vi "Error Handling Core.vi"(8 "error in (no error)":errorcluster) -> (0 "error out":errorcluster)   [LabVIEW 2016, in "System.lvlib"]
doc: "This is the core VI for error logging.\nWhen the error occurred, this VI will sned abort event to other processes."
uses:
  System.lvlib
  Controls/Control_Data Functions.ctl
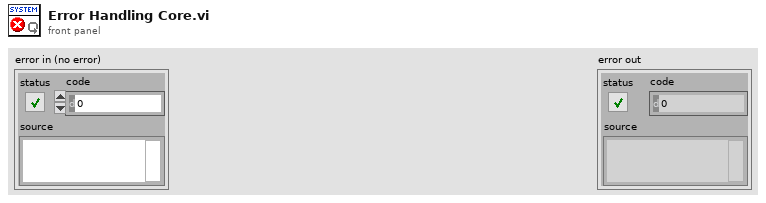
[diagram p1: front panel]
types:
  T1 = typedef "System.lvlib/Control_Data Functions.ctl" = enum16{"Get", "Set", "Release"}
  T2 = typedef "System.lvlib/Control_Queue Reference.ctl" = refnum<queue>
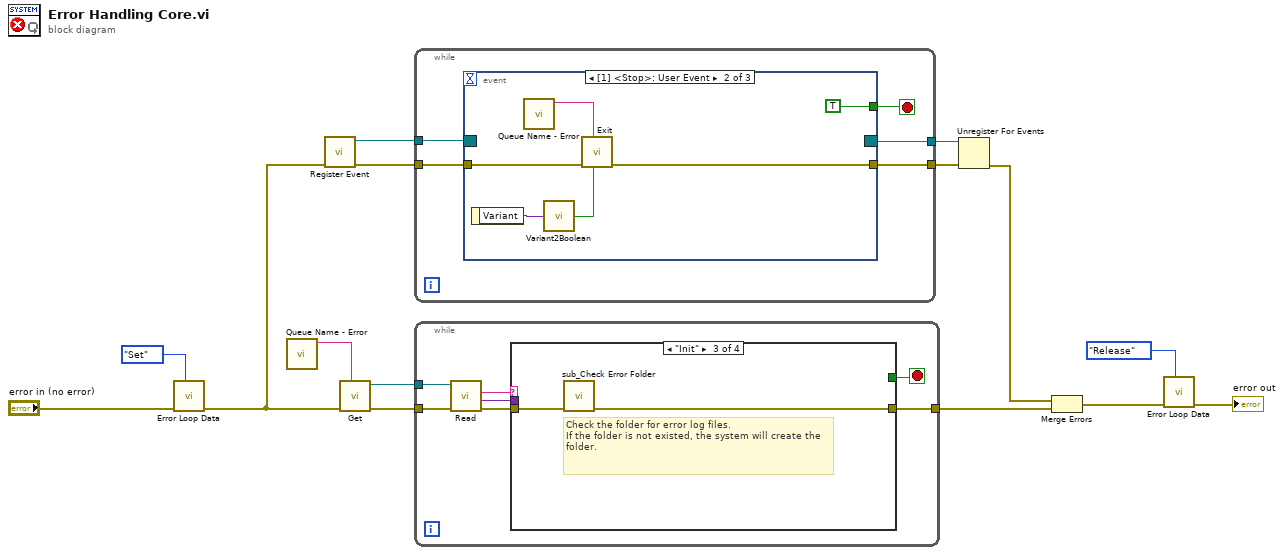
[diagram p0: block diagram]
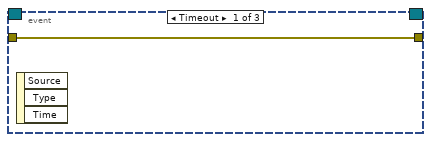
[diagram p2: hidden frame]
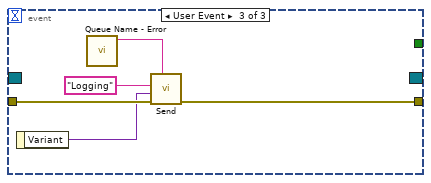
[diagram p3: hidden frame]
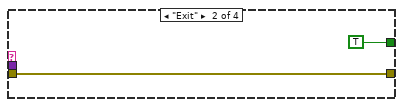
[diagram p5: hidden frame]
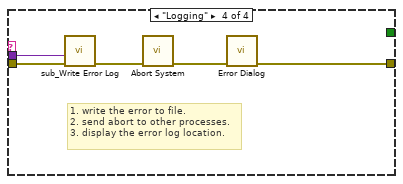
[diagram p6: hidden frame]
diagram:
  n1 = call "Error Loop Data.vi"("Data Functions"=Control_Data_Functions."Set", "error in (no error)"="error in (no error)") -> ("error out"=w10:errorcluster)  [unwired: 8 in, 1 out]
  n2 = call "Queue Name - Error.vi"() -> ("Process Name"=w15:string)  [unwired: 11 in]
  n3 = call "Register Event.vi"("error in (no error)"=w10) -> ("error out"=w12:errorcluster, "Event Registration Refnum"=w11:refnum<event-registration>)  [unwired: 9 in]
  n4 = call "Get.vi"("Process Name"=w15, "error in (no error)"=w10) -> ("error out"=w13:errorcluster, "queue out"=w14:T2)  [unwired: 8 in]
  n5 = while {
    tunnel: w12 -> [w20]
    tunnel: w11 -> [w19]
    tunnel: [w18] -> w2
    tunnel: [w16] -> w3
    stop <- w17 stop-if-true
    n6 = event shown="[1] <Stop>: User Event" {
      selector: w19 -> [_ _ _]
      dyn-events: [_ _ _] -> w16
      timeout: _ -> [_ _ _]
      tunnel: w20 -> [w21 w27 w32]
      tunnel: [w21 w25 w31] -> w18
      tunnel: [_ TRUE _] -> w17
      event Timeout {
        n7 = event-data() -> ()  [unwired: 1 in, 3 out]
      }
      event User Event {
        n8 = event-data() -> ("Variant"=w23:variant)  [unwired: 1 in]
        n9 = call "Queue Name - Error.vi"() -> ("Process Name"=w26:string)  [unwired: 11 in]
        n10 = call "Variant2Boolean.vi"("Data"=w23) -> ("Boolean"=w22:bool)  [unwired: 4 in]
        n11 = call "Exit.vi"("Priority (F)"=w22, "Process Name"=w26, "error in (no error)"=w27) -> ("error out"=w25:errorcluster)  [unwired: 8 in]
      }
      event User Event {
        n12 = event-data() -> ("Variant"=w28:variant)  [unwired: 1 in]
        n13 = call "Queue Name - Error.vi"() -> ("Process Name"=w30:string)  [unwired: 11 in]
        n14 = call "Send.vi"("Process Name"=w30, "error in (no error)"=w32, "Data"=w28, "Message"="Logging") -> ("error out"=w31:errorcluster)  [unwired: 7 in]
      }
    }
  }
  n15 = while {
    tunnel: w14 -> [w39]
    tunnel: w13 -> [w38]
    tunnel: [w34] -> w7
    stop <- w33 stop-if-true
    n16 = call "Read.vi"("error in (no error)"=w38, "queue out"=w39) -> ("error out"=w35:errorcluster, "Data"=w36:variant, "Message"=w37:string)  [unwired: 5 in, 2 out]
    n17 = case shown="\"Init\"" w37 {
      tunnel: w36 -> [_ _ _ w48]
      tunnel: w35 -> [w40 w42 w44 w49]
      tunnel: [w40 w42 w43 w45] -> w34
      tunnel: [_ TRUE _ _] -> w33
      frame Default {
      }
      frame "Exit" {
      }
      frame "Init" {
        # "Check the folder for error log files.\nIf the folder is not existed, the system will create the folder."
        n18 = call "sub_Check Error Folder.vi"("error in (no error)"=w44) -> ("error out"=w43:errorcluster)  [unwired: 10 in]
      }
      frame "Logging" {
        # "1. write the error to file.\n2. send abort to other processes.\n3. display the error log location."
        n19 = call "sub_Write Error Log.vi"("error in (no error)"=w49, "Data"=w48) -> ("error out"=w47:errorcluster)  [unwired: 9 in]
        n20 = call "Abort System.vi"("error in (no error)"=w47) -> ("error out"=w46:errorcluster)  [unwired: 10 in]
        n21 = call "Error Dialog.vi"("error in (no error)"=w46) -> ("error out"=w45:errorcluster)  [unwired: 10 in]
      }
    }
  }
  n22 = Unregister For Events(event registration refnum=w3, error in=w2) -> (error out=w1:errorcluster)
  n23 = Merge Errors(w1, w7) -> (w6:errorcluster)
  n24 = call "Error Loop Data.vi"("Data Functions"=Control_Data_Functions."Release", "error in (no error)"=w6) -> ("error out"=→"error out":errorcluster)  [unwired: 8 in, 1 out]
